vi "Drive_Hardware_Loop.vi"   [LabVIEW 2020]
uses:
  <vilib>/Rock Robotics/WPI/ThirdParty/Phoenix-LabVIEW/Motor Controller/Controls/CTRE_Phoenix_MotorControl_ControlMode.ctl
  Drive_Hardware_Globals.vi
  Globals/Drive_Globals.vi
panel:
  # "e"
types:
  T1 = typedef "WPI_MotorControlDeviceRef.ctl" = cluster{"DeviceStatus":errorcluster, "Type":T2, "PWM":cluster{"PWM Channel":T3, "DeadBand":T4}, "CAN":cluster{"Device Number":u8, "SetOutput VI Ref":variant, "GetOutput VI Ref":variant, "Enable VI Ref":variant, "Disable VI Ref":variant, "Data":variant}, "Invert":bool, "DIO PWM":cluster{"PWM \"Enable\" Channel":T3, "DIOChannel":T5, "PWM Rate":dbl}}
  T2 = typedef "WPI_MotorControlType.ctl" = enum16{"PWM", "CAN", "DIO PWM"}
  T3 = typedef "FPGA_DIOPWMChannel.ctl" = enum8{"PWM 0", "PWM 1", "PWM 2", "PWM 3", "PWM 4", "PWM 5", "PWM 6", "PWM 7", "PWM 8", "PWM 9", "PWM MXP 0", "PWM MXP 1", "PWM MXP 2", "PWM MXP 3", "PWM MXP 4", "PWM MXP 5", "PWM MXP 6", "PWM MXP 7", "PWM MXP 8", "PWM MXP 9", "Invalid"}
  T4 = typedef "WPI_PWMDeadband.ctl" = cluster{"Name":string, "maxPositivePwm":i32, "minPositivePwm":i32, "centerPwm":i32, "maxNegativePwm":i32, "minNegativePwm":i32, "angularRange":u16}
  T5 = typedef "FPGA_DIOChannel.ctl" = enum8{"DIO 0", "DIO 1", "DIO 2", "DIO 3", "DIO 4", "DIO 5", "DIO 6", "DIO 7", "DIO 8", "DIO 9", "DIO MXP 0", "DIO MXP 1", "DIO MXP 2", "DIO MXP 3", "DIO MXP 4", "DIO MXP 5", "DIO MXP 6", "DIO MXP 7", "DIO MXP 8", "DIO MXP 9", "DIO MXP 10", "DIO MXP 11", "DIO MXP 12", "DIO MXP 13", "DIO MXP 14", "DIO MXP 15", "SPI Port CS1", "SPI Port CS2", "SPI Port CS3", "SPI Port MISO", "SPI Port MOSI", "Invalid"}
  T6 = typedef "CTRE_Phoenix_MotorControl_ControlMode.ctl" = u16
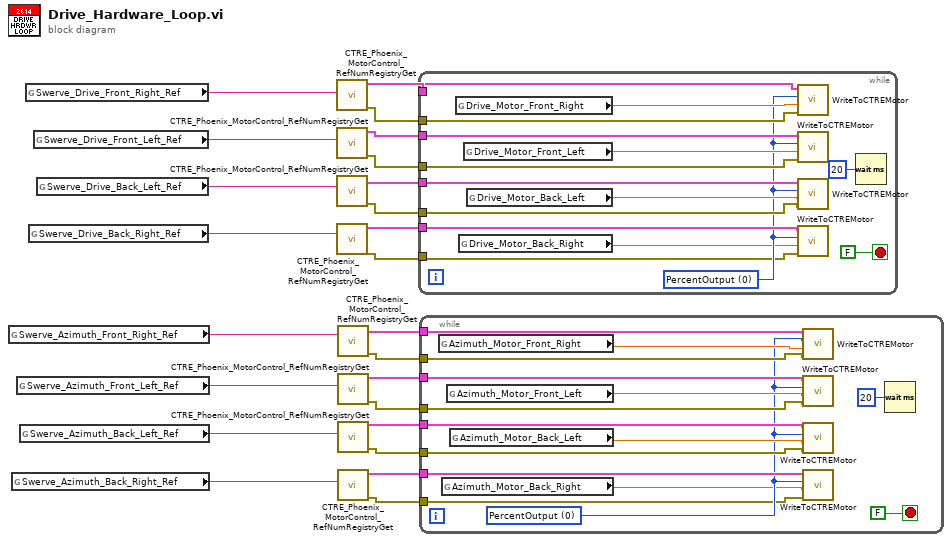
[diagram p0: block diagram]
diagram:
  n1 = global read "Drive_Hardware_Globals.vi" "Swerve_Azimuth_Front_Right_Ref"() -> (w4:string)
  n2 = global read "Drive_Hardware_Globals.vi" "Swerve_Azimuth_Back_Right_Ref"() -> (w1:string)
  n3 = global read "Drive_Hardware_Globals.vi" "Swerve_Azimuth_Front_Left_Ref"() -> (w3:string)
  n4 = global read "Drive_Hardware_Globals.vi" "Swerve_Azimuth_Back_Left_Ref"() -> (w2:string)
  n5 = global read "Drive_Hardware_Globals.vi" "Swerve_Drive_Front_Right_Ref"() -> (w8:string)
  n6 = global read "Drive_Hardware_Globals.vi" "Swerve_Drive_Back_Right_Ref"() -> (w5:string)
  n7 = global read "Drive_Hardware_Globals.vi" "Swerve_Drive_Front_Left_Ref"() -> (w7:string)
  n8 = global read "Drive_Hardware_Globals.vi" "Swerve_Drive_Back_Left_Ref"() -> (w6:string)
  n9 = call <vilib>:"CTRE_Phoenix_MotorControl_RefNumRegistryGet.vi"("refnum name"=w8) -> ("error out"=w16:errorcluster, "PhoenixMotorControlDevRef"=w17:T1)  [unwired: 9 in]
  n10 = call <vilib>:"CTRE_Phoenix_MotorControl_RefNumRegistryGet.vi"("refnum name"=w7) -> ("error out"=w15:errorcluster, "PhoenixMotorControlDevRef"=w18:T1)  [unwired: 9 in]
  n11 = call <vilib>:"CTRE_Phoenix_MotorControl_RefNumRegistryGet.vi"("refnum name"=w6) -> ("error out"=w14:errorcluster, "PhoenixMotorControlDevRef"=w19:T1)  [unwired: 9 in]
  n12 = call <vilib>:"CTRE_Phoenix_MotorControl_RefNumRegistryGet.vi"("refnum name"=w5) -> ("error out"=w13:errorcluster, "PhoenixMotorControlDevRef"=w20:T1)  [unwired: 9 in]
  n13 = call <vilib>:"CTRE_Phoenix_MotorControl_RefNumRegistryGet.vi"("refnum name"=w4) -> ("error out"=w12:errorcluster, "PhoenixMotorControlDevRef"=w21:T1)  [unwired: 9 in]
  n14 = call <vilib>:"CTRE_Phoenix_MotorControl_RefNumRegistryGet.vi"("refnum name"=w3) -> ("error out"=w11:errorcluster, "PhoenixMotorControlDevRef"=w22:T1)  [unwired: 9 in]
  n15 = call <vilib>:"CTRE_Phoenix_MotorControl_RefNumRegistryGet.vi"("refnum name"=w2) -> ("error out"=w10:errorcluster, "PhoenixMotorControlDevRef"=w23:T1)  [unwired: 9 in]
  n16 = call <vilib>:"CTRE_Phoenix_MotorControl_RefNumRegistryGet.vi"("refnum name"=w1) -> ("error out"=w9:errorcluster, "PhoenixMotorControlDevRef"=w24:T1)  [unwired: 9 in]
  n17 = while {
    tunnel: w20 -> [w28]
    tunnel: w19 -> [w29]
    tunnel: w18 -> [w34]
    tunnel: w17 -> [w37]
    tunnel: w16 -> [w35]
    tunnel: w15 -> [w32]
    tunnel: w14 -> [w30]
    tunnel: w13 -> [w25]
    stop <- FALSE stop-if-true
    w27 = T6 0 items=["PercentOutput"=0, "Position"=1, "Velocity"=2, "Current"=3, "Follower"=5, "MotionProfile"=6, "MotionMagic"=7, "MotionProfileArc"=10, "Disabled"=15] ("Control Mode")
    n18 = global read "Drive_Globals.vi" "Drive_Motor_Front_Right"() -> (w36:dbl)
    n19 = global read "Drive_Globals.vi" "Drive_Motor_Back_Right"() -> (w26:dbl)
    n20 = global read "Drive_Globals.vi" "Drive_Motor_Front_Left"() -> (w33:dbl)
    n21 = global read "Drive_Globals.vi" "Drive_Motor_Back_Left"() -> (w31:dbl)
    n22 = call "WriteToCTREMotor.vi"("error in (no error)"=w35, "Motor_Value"=w36, "Control Mode"=w27, "PhoenixMotorControlDevRef"=w37) -> ()  [unwired: 8 in]
    n23 = call "WriteToCTREMotor.vi"("error in (no error)"=w32, "Motor_Value"=w33, "Control Mode"=w27, "PhoenixMotorControlDevRef"=w34) -> ()  [unwired: 8 in]
    n24 = call "WriteToCTREMotor.vi"("error in (no error)"=w30, "Motor_Value"=w31, "Control Mode"=w27, "PhoenixMotorControlDevRef"=w29) -> ()  [unwired: 8 in]
    n25 = call "WriteToCTREMotor.vi"("error in (no error)"=w25, "Motor_Value"=w26, "Control Mode"=w27, "PhoenixMotorControlDevRef"=w28) -> ()  [unwired: 8 in]
    n26 = Wait (ms)(milliseconds to wait=u32 20) -> ()  [unwired: 1 out]
  }
  n27 = while {
    tunnel: w24 -> [w43]
    tunnel: w23 -> [w46]
    tunnel: w22 -> [w49]
    tunnel: w21 -> [w52]
    tunnel: w12 -> [w50]
    tunnel: w11 -> [w47]
    tunnel: w10 -> [w44]
    tunnel: w9 -> [w40]
    stop <- FALSE stop-if-true
    w42 = T6 0 items=["PercentOutput"=0, "Position"=1, "Velocity"=2, "Current"=3, "Follower"=5, "MotionProfile"=6, "MotionMagic"=7, "MotionProfileArc"=10, "Disabled"=15] ("Control Mode")
    n28 = global read "Drive_Globals.vi" "Azimuth_Motor_Front_Right"() -> (w51:dbl)
    n29 = global read "Drive_Globals.vi" "Azimuth_Motor_Back_Right"() -> (w41:dbl)
    n30 = global read "Drive_Globals.vi" "Azimuth_Motor_Front_Left"() -> (w48:dbl)
    n31 = global read "Drive_Globals.vi" "Azimuth_Motor_Back_Left"() -> (w45:dbl)
    n32 = call "WriteToCTREMotor.vi"("error in (no error)"=w50, "Motor_Value"=w51, "Control Mode"=w42, "PhoenixMotorControlDevRef"=w52) -> ()  [unwired: 8 in]
    n33 = call "WriteToCTREMotor.vi"("error in (no error)"=w47, "Motor_Value"=w48, "Control Mode"=w42, "PhoenixMotorControlDevRef"=w49) -> ()  [unwired: 8 in]
    n34 = call "WriteToCTREMotor.vi"("error in (no error)"=w44, "Motor_Value"=w45, "Control Mode"=w42, "PhoenixMotorControlDevRef"=w46) -> ()  [unwired: 8 in]
    n35 = call "WriteToCTREMotor.vi"("error in (no error)"=w40, "Motor_Value"=w41, "Control Mode"=w42, "PhoenixMotorControlDevRef"=w43) -> ()  [unwired: 8 in]
    n36 = Wait (ms)(milliseconds to wait=u32 20) -> ()  [unwired: 1 out]
  }
